vi "KepcoDCPwr Reset Output Protection.vi"(0 "VISA Session":refnum<visa-resource-name>, 5 "Model In":string, 7 "channel name (\"\")":string="\"\"", 11 "error in (no error)":errorcluster {"code" format="%.0x"}) -> (4 "VISA Session Out":refnum<visa-resource-name>, 6 "Model Out":string, 8 "channel name out (\"\")":string="\"\"" caption="channel name Out (\"\")", 15 "error out":errorcluster {"code" format="%.0x"})   [LabVIEW 2010]
doc: "This VI resets the power supply's output protection after an over-voltage, over-current, or other output protection condition occurs.\n\nAn over-voltage condition occurs when the output voltage is equal to or greater than the value of the OVP Limit property and the OVP Enabled property is set to TRUE. \n\n\nWhen either an over-voltage condition or an over-current condition occurs, the output protection of the power supply disables the output. Once the output protection is reset, the power supply resumes generating a power signal.\n\nYou use the KepcoDCPwr Query Output State.vi to determine if the power supply is in an output-protection state."
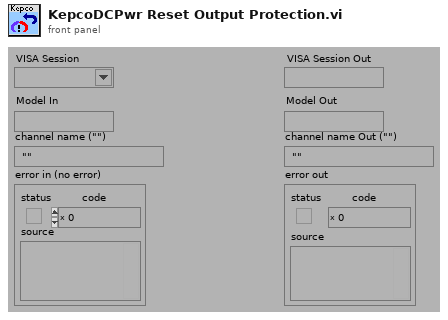
[diagram p1: front panel]
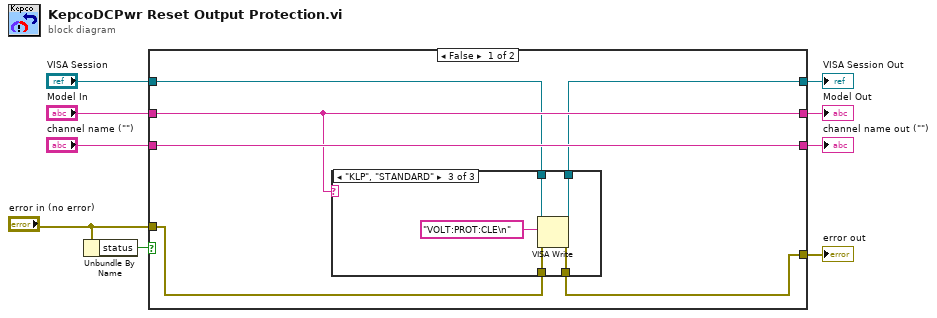
[diagram p0: block diagram]
diagram:
  n1 = Unbundle By Name("error in (no error)") -> ("status"=w8:bool)
  n2 = case shown="False" w8 {
    tunnel: [w11 w28] -> w9
    tunnel: "error in (no error)" -> [w10 w28]
    tunnel: [w12 w27] -> w3
    tunnel: "VISA Session" -> [w13 w27]
    tunnel: [w14 w26] -> w2
    tunnel: "Model In" -> [w14 w26]
    tunnel: [w15 w25] -> w1
    tunnel: "channel name (\"\")" -> [w15 w25]
    frame False {
      n3 = case shown="\"KLP\", \"STANDARD\"" w14 {
        tunnel: w10 -> [w16 w18 w23]
        tunnel: w13 -> [w17 w19 w22]
        tunnel: [w17 w19 w21] -> w12
        tunnel: [w16 w18 w20] -> w11
        frame "", Default {
        }
        frame "BOP-HP", "BOP-LP", "MULTI", "MULTI_PLUS" {
        }
        frame "KLP", "STANDARD" {
          n4 = VISA Write(VISA resource name=w22, write buffer="VOLT:PROT:CLE\n", error in (no error)=w23) -> (VISA resource name out=w21:refnum<visa-resource-name>, error out=w20:errorcluster)  [unwired: 1 out]
        }
      }
    }
    frame True {
    }
  }
  "error out" <- w9
  "channel name out (\"\")" <- w1
  "Model Out" <- w2
  "VISA Session Out" <- w3
